vi "Panel.vi"(6 "Fiber Auto Collimation state data":refnum<class "Fiber Auto Collimation state data.lvclass">, 7 "Station config":refnum<class "Station config.lvclass">, 8 "error in (no error)":errorcluster, 11 "Fiber Auto Collimation panel in":refnum<class "Fiber Auto Collimation panel.lvclass">) -> (0 "error out":errorcluster, 3 "Fiber Auto Collimation panel out":refnum<class "Fiber Auto Collimation panel.lvclass">)   [LabVIEW 2018, in "Fiber Auto Collimation panel.lvclass"]
doc: "This VI is not functional by itself but is there to be inherited by any descendant class of the top-level Panel class. It is highly recommended to create a new Panel class by copying an existing one instead of a new one because of the long list of required responsibilities of a Panel VI. These responsibilities are listed as comments on the block diagram of this top level VI if it is being created fresh instead of copied from a template.\n\nNote that this VI needs to remain reentrant to be compatible with all other Panel classes that might want multiple instances of themselves to be open at once. \n\nAlso note that the appearance of this window is not set to open when it runs. This is because the panel launcher has an option to start any panel hidden, so the \"Register panel as running\" VI that executes later can set it to appear or not as needed."
uses:
  Fiber Auto Collimation panel.lvclass
  State data/Fiber Auto Collimation state data.lvclass
  <userlib>/Recipe/Station Config/Station config.lvclass
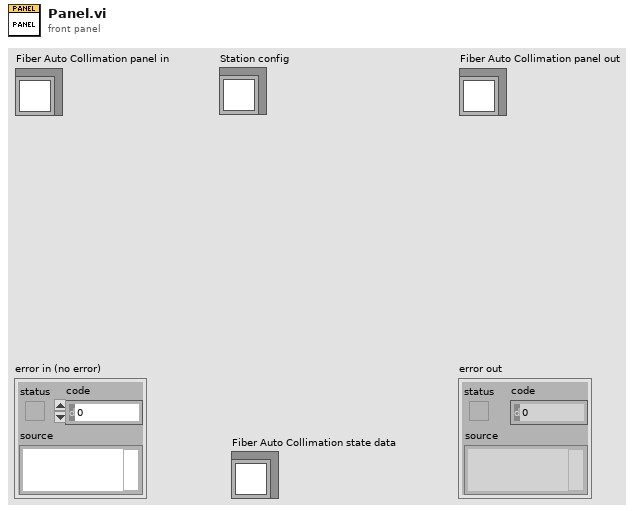
[diagram p1: front panel]
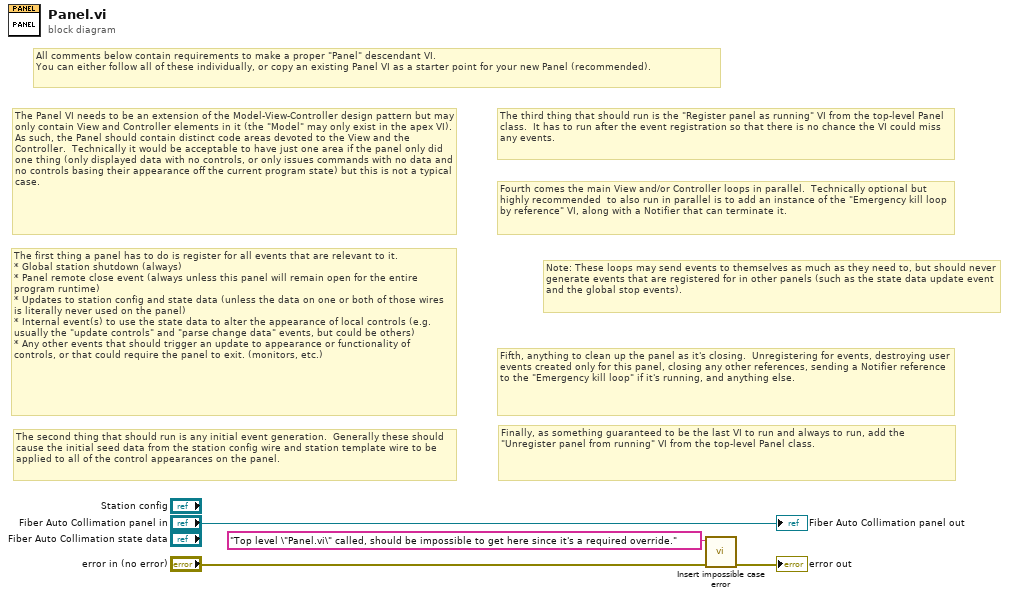
[diagram p0: block diagram]
diagram:
  # "Finally, as something guaranteed to be the last VI to run and always to run, add the \"Unregister panel from running\" VI from the top-level Panel class."
  # "Fifth, anything to clean up the panel as it's closing.  Unregistering for events, destroying user events created only for this panel, closing any other references, sending a Notifier reference to the \"Emergency kill loop\" if it's running, and anything else."
  # "Fourth comes the main View and/or Controller loops in parallel.  Technically optional but highly recommended  to also run in parallel is to add an instance of the \"Emergency kill loop by reference\" VI, along with a Notifier that can terminate it."
  # "The third thing that should run is the \"Register panel as running\" VI from the top-level Panel class.  It has to run after the event registration so that there is no chance the VI could miss any events."
  # "Note: These loops may send events to themselves as much as they need to, but should never generate events that are registered for in other panels (such as the state data update event and the global stop events)."
  # "The second thing that should run is any initial event generation.  Generally these should cause the initial seed data from the station config wire and station template wire to be applied to all of the control appearances on the panel."
  # "The first thing a panel has to do is register for all events that are relevant to it.\n* Global station shutdown (always)\n* Panel remote close event (always unless this panel will remain open for the entire program runtime)\n* Updates to station config and state data (unless the data on one or both of those wires is literally never used on the panel)\n* Internal event(s) to use the state data to alter the appearance of local controls (e.g. usually the \"update controls\" and \"parse change data\" events, but could be others)\n* Any other events that should trigger an update to appearance or functionality of controls, or that could require the panel to exit. (monitors, etc.)"
  # "The Panel VI needs to be an extension of the Model-View-Controller design pattern but may only contain View and Controller elements in it (the \"Model\" may only exist in the apex VI).\nAs such, the Panel should contain distinct code areas devoted to the View and the Controller.  Technically it would be acceptable to have just one area if the panel only did one thing (only displayed data with no controls, or only issues commands with no data and no controls basing their appearance off the current program state) but this is not a typical case."
  # "All comments below contain requirements to make a proper \"Panel\" descendant VI.  \nYou can either follow all of these individually, or copy an existing Panel VI as a starter point for your new Panel (recommended)."
  n1 = call <userlib>:"Insert impossible case error.vi"("error in (no error)"="error in (no error)", "Optional extra info"="Top level \"Panel.vi\" called, should be impossible to get here since it's a required override.") -> ("error out"=→"error out":errorcluster)  [unwired: 9 in]
  "Fiber Auto Collimation panel out" <- "Fiber Auto Collimation panel in"
